vi "Get Windows Primary Language.vi"() -> (2 "Primary Language":string)   [LabVIEW 2017, in "JKI Simple Localization.lvlib"]
doc: "Query windows to identify the OSs primary language"
uses:
  API/JKI Simple Localization.lvlib
  kernel32.dll
panel:
  out "Primary Language Ring Control":u16(ring) items=["Swahili"=65, "Malay"=62, "Faeroese"=56, "Afrikaans"=54, "Basque"=45, "Farsi"=41, "Lithuanian"=39, "Latvian"=38, "Estonian"=37, "Slovenian"=36, "Belarusian"=35, "Ukrainian"=34, "Indonesian"=33, "Turkish"=31, "Thai"=30, "Swedish"=29, "Albanian"=28, "Slovak"=27, "Serbo-Croatian"=26, "Russian"=25, "Romanian"=24, "Portuguese"=22, "Polish"=21, "Norwegian"=20, "Dutch"=19, "Korean"=18, "Japanese"=17, "Italian"=16, "Icelandic"=15, "Hungarian"=14, "Hebrew"=13, "French"=12, "Finnish"=11, "Spanish"=10, "English"=9, "Greek"=8, "German"=7, "Danish"=6, "Czech"=5, "Chinese"=4, "Catalan"=3, "Bulgarian"=2, "Arabic"=1]
  out "Default Language Identifier":u32 format="%.0x"
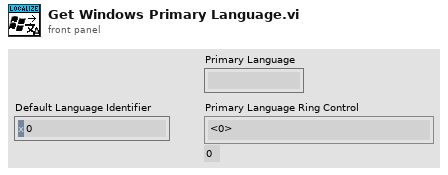
[diagram p1: front panel]
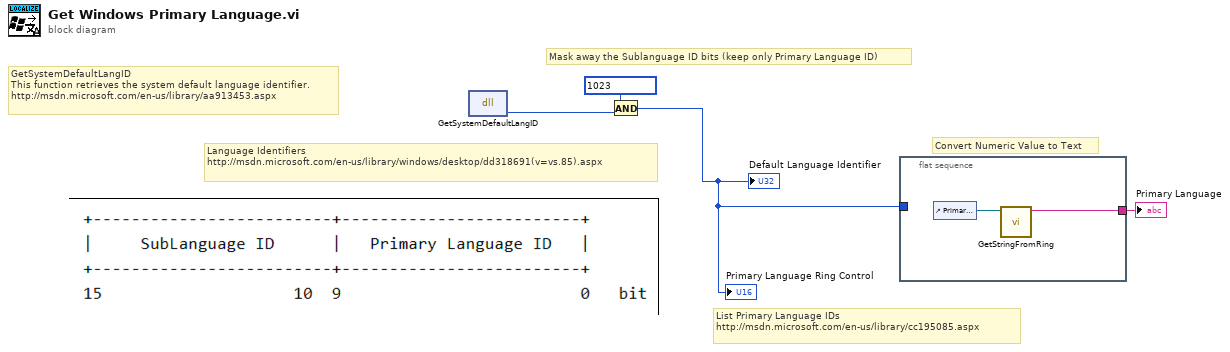
[diagram p0: block diagram]
diagram:
  # "Convert Numeric Value to Text"
  # "Mask away the Sublanguage ID bits (keep only Primary Language ID)"
  # "List Primary Language IDs\nhttp://msdn.microsoft.com/en-us/library/cc195085.aspx"
  # "GetSystemDefaultLangID\nThis function retrieves the system default language identifier.\nhttp://msdn.microsoft.com/en-us/library/aa913453.aspx"
  # "Language Identifiers\nhttp://msdn.microsoft.com/en-us/library/windows/desktop/dd318691(v=vs.85).aspx"
  n1 = dll-call lib="kernel32.dll" fn="GetSystemDefaultLangID" label="kernel32.dll\nGetSystemDefaultLangID"() -> ("return type"=w2:u16)  [unwired: 3 in, 2 out]
  n2 = And(x=u16 1023 ("return type"), y=w2) -> (x .and. y?=w1:u16)
  "Default Language Identifier" <- w1
  "Primary Language Ring Control" <- w1
  n3 = flat-sequence {
    tunnel: w1 -> [_]
    tunnel: [w5] -> w4
    frame #0 {
      n4 = control-ref of="Primary Language Ring Control"() -> (w6:refnum<vi>)
      n5 = call "GetStringFromRing.vi"("Ring Reference"=w6) -> ("String"=w5:string)  [unwired: 9 in, 1 out]
    }
  }
  "Primary Language" <- w4
